vi "setTrigger.vi"(8 "error in":errorcluster, 9 "Trigger Settings":T3={"DC Restore"=enum."off", "Polarity"=enum."Negative", "TV Event"=enum."Field 1", "Coupling"=enum."AC", "Slope"=enum."Negative", "AnalogSource"=enum."Channel 0", "Window Mode"=enum."Entering", "Low Level"=0.0, "High Level"=0.0, "Hysteresis"=0.0, "Delay"=0.0, "Holdoff"=0.0, "Signal Format"=enum."M-NTSC", "Mode"=enum."Immediate", "Line Number"=0, "DigitalSource"=enum."RTSI 0"}, 11 "instrument handle":refnum<k15>) -> (0 "error out":errorcluster, 1 "Trigger Settings out":T3={"DC Restore"=enum."off", "Polarity"=enum."Negative", "TV Event"=enum."Field 1", "Coupling"=enum."AC", "Slope"=enum."Negative", "AnalogSource"=enum."Channel 0", "Window Mode"=enum."Entering", "Low Level"=0.0, "High Level"=0.0, "Hysteresis"=0.0, "Delay"=0.0, "Holdoff"=0.0, "Signal Format"=enum."M-NTSC", "Mode"=enum."Immediate", "Line Number"=0, "DigitalSource"=enum."RTSI 0"}, 3 "instrument handle out":refnum<k15>)   [LabVIEW 2011]
uses:
  niScope trigger source.ctl
  niScope trigger source digital.ctl
  TriggerSettings_TypDef.ctl
  OnOffTypeDef.ctl
  Polarity_TypDEf.ctl
  TVEvent_TypDef.ctl
  coupling_TypDef.ctl
  positive_negatice2_typDef.ctl
  TriggerSource_TypDef.ctl
  triggerwindowmode2_TypDef.ctl
  SignalFormat_TypDef.ctl
  mode_TypDef.ctl
  Trigger.DigitalSource_TypDEf.ctl
  LVStringsAndValuesArrayTypeDef.ctl
panel:
  in  "Trigger Source window 2":T1="0" caption="Source"
  out "Channel Selection out":string
  out "Mode":T2
  in  "trigger source (dig)":T13="VAL_RTSI_0" caption="trigger source (RTSI 0)"
  in  "Trigger Source Video 2":T1="0" caption="Source"
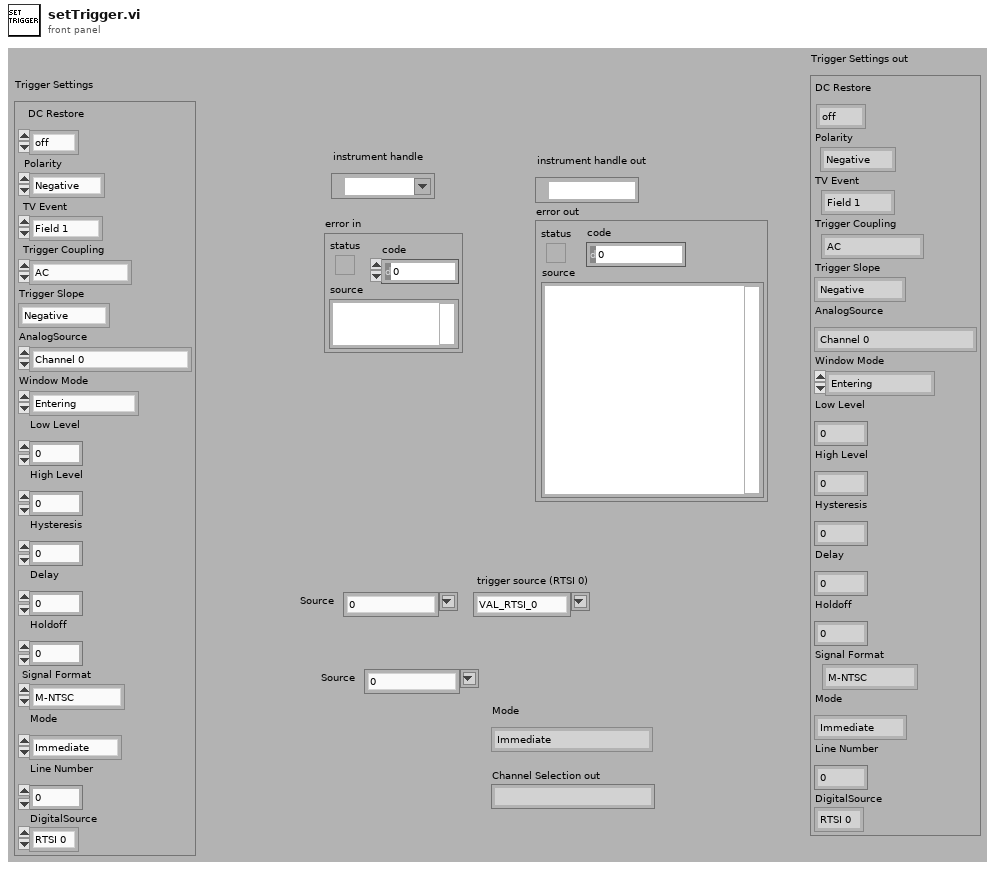
[diagram p1: front panel]
types:
  T1 = typedef "niScope trigger source.ctl" = string
  T2 = typedef "mode_TypDef.ctl" = enum32{"Immediate", "Analog Edge", "Analog Window", "Analog Hysteresis", "Video", "Digital Edge"}
  T3 = typedef "TriggerSettings_TypDef.ctl" = cluster{"DC Restore":T4, "Polarity":T5, "TV Event":T6, "Coupling":T7, "Slope":T8, "AnalogSource":T9, "Window Mode":T10, "Low Level":dbl, "High Level":dbl, "Hysteresis":dbl, "Delay":dbl, "Holdoff":dbl, "Signal Format":T11, "Mode":T2, "Line Number":i32, "DigitalSource":T12}
  T4 = typedef "OnOffTypeDef.ctl" = enum16{"off", "on"}
  T5 = typedef "Polarity_TypDEf.ctl" = enum16{"Negative", "Positive"}
  T6 = typedef "TVEvent_TypDef.ctl" = enum16{"Field 1", "Field 2", "Any Field", "Any Line", "Line Number"}
  T7 = typedef "coupling_TypDef.ctl" = enum16{"AC", "DC", "HF Reject", "LF Reject", "AC Plus HF Reject"}
  T8 = typedef "positive_negatice2_typDef.ctl" = enum16{"Positive", "Negative"}
  T9 = typedef "TriggerSource_TypDef.ctl" = enum16{"Channel 0", "Channel 1", "External TRIG"}
  T10 = typedef "triggerwindowmode2_TypDef.ctl" = enum16{"Entering", "Leaving"}
  T11 = typedef "SignalFormat_TypDef.ctl" = enum16{"M-NTSC", "B/G-PAL", "SECAM", "M-PAL", "480i/59.94 fps", "480i/60 fps", "480p/59.94 Fps", "480p/60 Fps", "576i/50 fps", "576p/50 Fps", "720p/50 Fps", "720p/59.94 Fps", "720p/60 Fps", "1080i/50 fps", "1080i/59.94 fps", "1080i/60 fps", "1080p/24 Fps"}
  T12 = typedef "Trigger.DigitalSource_TypDEf.ctl" = enum16{"RTSI 0", "RTSI 1", "RTSI 2", "RTSI 3", "RTSI 4", "RTSI 5", "RTSI 6", "PFI 0", "PFI 1", "PFI 2", "PXI Star Trigger"}
  T13 = typedef "niScope trigger source digital.ctl" = string
  T14 = typedef "LVStringsAndValuesArrayTypeDef.ctl" = cluster{"String":string, "Value":ext}[]
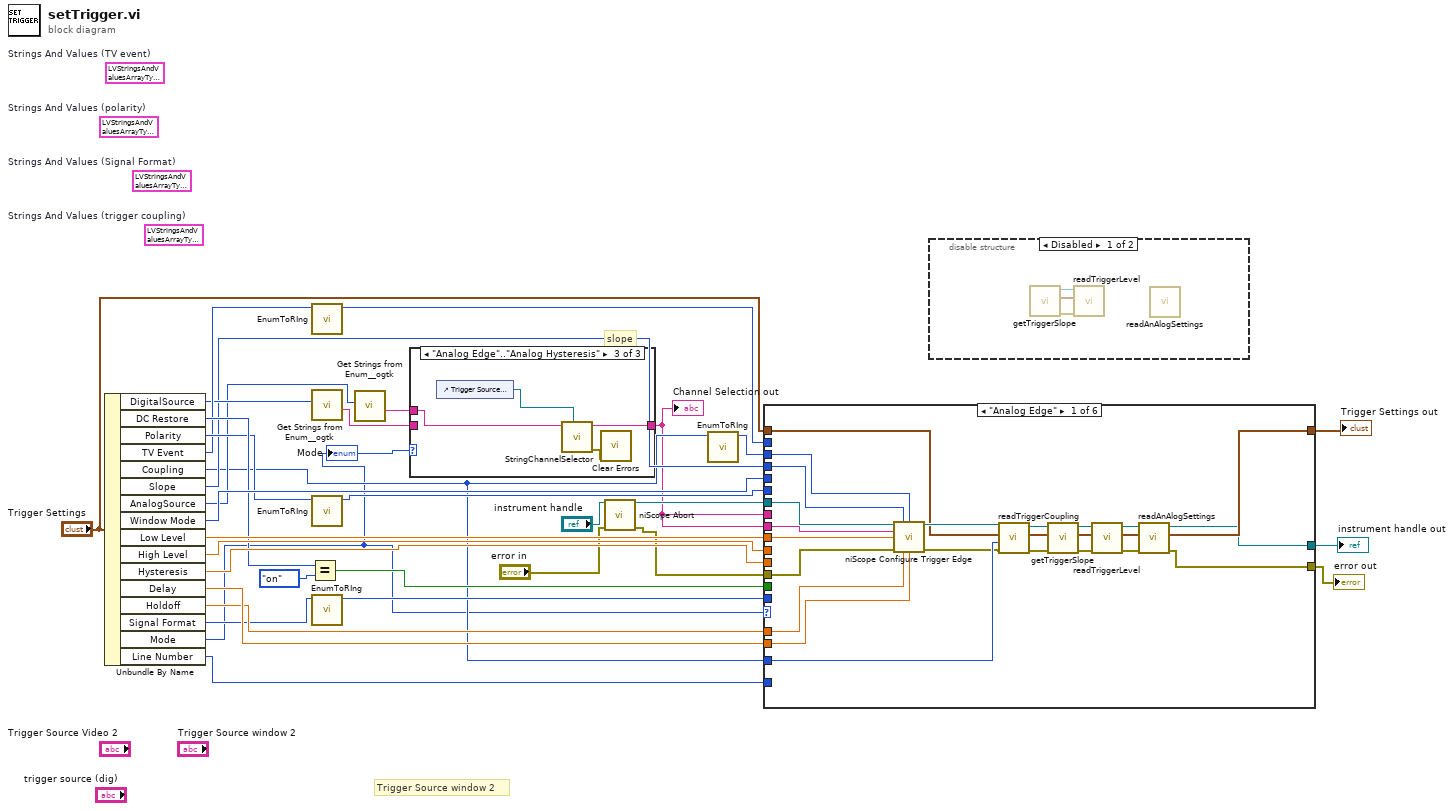
[diagram p0: block diagram]
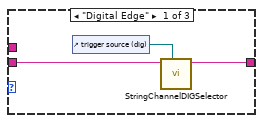
[diagram p3: hidden frame]
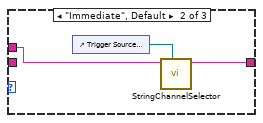
[diagram p4: hidden frame]
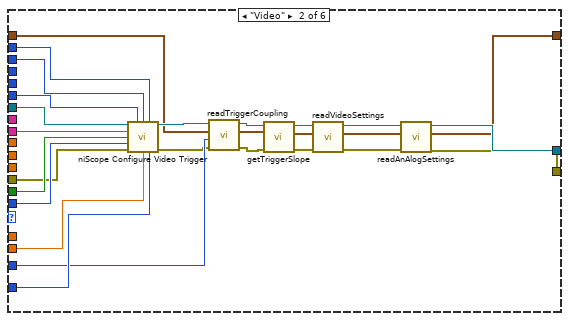
[diagram p5: hidden frame]
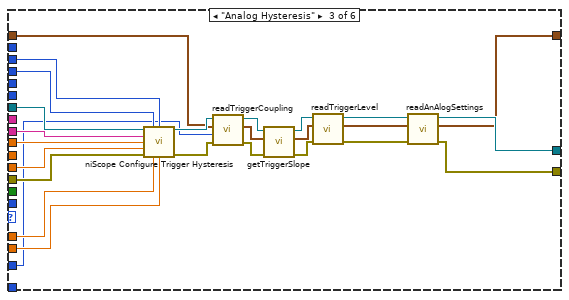
[diagram p6: hidden frame]
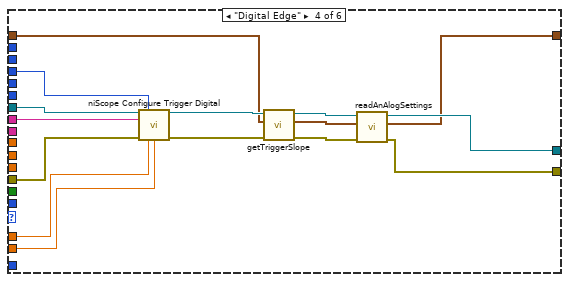
[diagram p7: hidden frame]
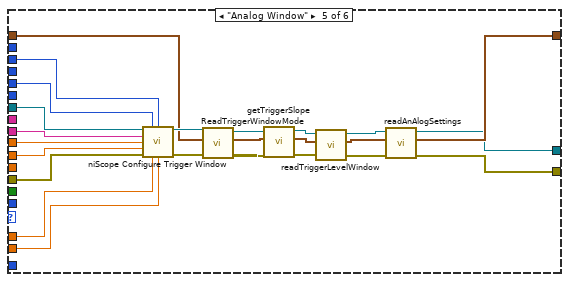
[diagram p8: hidden frame]
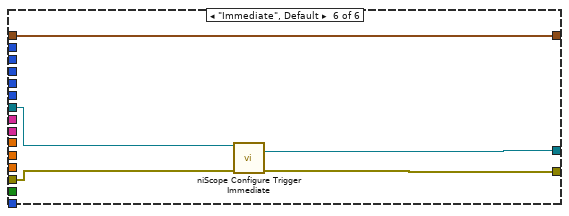
[diagram p9: hidden frame]
diagram:
  (unwired) T14 [{"String"="M-NTSC", "Value"=1.0}, {"String"="B/G-PAL", "Value"=2.0}, {"String"="SECAM", "Value"=3.0}, {"String"="M-PAL", "Value"=1001.0}, {"String"="480i/59.94 fps", "Value"=1010.0}, {"String"="480i/60 fps", "Value"=1011.0}, {"String"="480p/59.94 Fps", "Value"=1015.0}, {"String"="480p/60 Fps", "Value"=1016.0}, {"String"="576i/50 fps", "Value"=1020.0}, {"String"="576p/50 Fps", "Value"=1025.0}, {"String"="720p/50 Fps", "Value"=1031.0}, {"String"="720p/59.94 Fps", "Value"=1032.0}, {"String"="720p/60 Fps", "Value"=1033.0}, {"String"="1080i/50 fps", "Value"=1040.0}, {"String"="1080i/59.94 fps", "Value"=1041.0}, {"String"="1080i/60 fps", "Value"=1042.0}, {"String"="1080p/24 Fps", "Value"=1045.0}]  # Strings And Values (Signal Format)
  (unwired) T14 [{"String"="Field 1", "Value"=1.0}, {"String"="Field 2", "Value"=2.0}, {"String"="Any Field", "Value"=3.0}, {"String"="Any Line", "Value"=4.0}, {"String"="Line Number", "Value"=5.0}]  # Strings And Values (TV event)
  (unwired) T14 [{"String"="Positive", "Value"=1.0}, {"String"="Negative", "Value"=2.0}]  # Strings And Values (polarity)
  (unwired) T14 [{"String"="AC", "Value"=0.0}, {"String"="DC", "Value"=1.0}, {"String"="HF Reject", "Value"=3.0}, {"String"="LF Reject", "Value"=4.0}, {"String"="AC Plus HF Reject", "Value"=1001.0}]  # Strings And Values (trigger coupling)
  # "Trigger Source window 2"
  # "slope"
  n1 = Unbundle By Name("Trigger Settings") -> ("DigitalSource"=w15:T12, "DC Restore"=w26:T4, "Polarity"=w18:T5, "TV Event"=w17:T6, "Coupling"=w7:T7, "Slope"=w11:T8, "AnalogSource"=w8:T9, "Window Mode"=w33:T10, "Low Level"=w32:dbl, "High Level"=w31:dbl, "Hysteresis"=w30:dbl, "Delay"=w29:dbl, "Holdoff"=w28:dbl, "Signal Format"=w16:T11, "Mode"=w5:T2, "Line Number"=w27:i32)
  "Mode" <- w5
  n2 = Equal?(x=w26, y=OnOffTypeDef."on" ("DC Restore")) -> (x = y?=w24:bool)
  n3 = call "EnumToRIng.vi"("Enum"=w17) -> ("Ring (Value)"=w21:u16)  [unwired: 10 in]
  n4 = call "Get Strings from Enum__ogtk.vi"("Enum"=w15) -> ("String Value"=w14:string)  [unwired: 7 in, 3 out]
  n5 = call "EnumToRIng.vi"("Enum"=w18) -> ("Ring (Value)"=w22:u16)  [unwired: 10 in]
  n6 = call "EnumToRIng.vi"("Enum"=w16) -> ("Ring (Value)"=w19:u16)  [unwired: 10 in]
  n7 = call "Get Strings from Enum__ogtk.vi"("Enum"=w8) -> ("String Value"=w23:string)  [unwired: 7 in, 3 out]
  n8 = case shown="\"Analog Edge\"..\"Analog Hysteresis\"" w5 {
    tunnel: [w35 w38 w43] -> w3
    tunnel: w23 -> [_ w37 w42]
    tunnel: w14 -> [w34 _ _]
    frame "Digital Edge" {
      n9 = control-ref of="trigger source (dig)"() -> (w36:refnum<vi>)
      n10 = call "StringChannelDIGSelector.vi"("ComboBoxREF"=w36, "input string"=w34) -> ("trigger source (dig)"=w35:T13)  [unwired: 8 in, 1 out]
    }
    frame "Immediate", Default {
      n11 = control-ref of="Trigger Source Video 2"() -> (w39:refnum<vi>)
      n12 = call "StringChannelSelector.vi"("reference 2"=w39, "input string"=w37) -> ("Channel Selection out"=w38:string)  [unwired: 8 in, 1 out]
    }
    frame "Analog Edge".."Analog Hysteresis" {
      n13 = control-ref of="Trigger Source window 2"() -> (w41:refnum<vi>)
      n14 = call "StringChannelSelector.vi"("reference 2"=w41, "input string"=w42) -> ("error out"=w40:errorcluster, "Channel Selection out"=w43:string)  [unwired: 8 in]
      n15 = call "Clear Errors.vi"("error in (no error)"=w40) -> ()  [unwired: 6 in, 1 out]
    }
  }
  "Channel Selection out" <- w3
  n16 = call "niScope Abort.vi"("instrument handle"="instrument handle", "error in"="error in") -> ("instrument handle out"=w12:refnum<k15>, "error out"=w1:errorcluster)  [unwired: 12 in]
  n17 = call "EnumToRIng.vi"("Enum"=w7) -> ("Ring (Value)"=w20:u16)  [unwired: 10 in]
  n18 = case "Trigger Selection" shown="\"Analog Edge\"" w5 {
    tunnel: [w46 w68 w94 w119 w146 w161] -> w6
    tunnel: [w58 w72 w108 w121 w147 w162] -> w10
    tunnel: w29 -> [w67 w93 w118 w133 w157 _]
    tunnel: w20 -> [w66 w92 w117 _ w156 _]
    tunnel: w11 -> [w57 _ w116 w132 _ _]
    tunnel: w32 -> [w61 _ w115 _ w155 _]
    tunnel: w3 -> [w65 w91 w114 _ w154 _]
    tunnel: w3 -> [_ _ _ w131 _ _]
    tunnel: w12 -> [w64 w90 w113 w130 w153 w160]
    tunnel: w28 -> [w63 _ w112 w129 w152 _]
    tunnel: w31 -> [_ _ _ _ w151 _]
    tunnel: w33 -> [_ _ _ _ w150 _]
    tunnel: w21 -> [_ w84 _ _ _ _]
    tunnel: w22 -> [_ w89 _ _ _ _]
    tunnel: w24 -> [_ w88 _ _ _ _]
    tunnel: w19 -> [_ w87 _ _ _ _]
    tunnel: w27 -> [_ w86 _ _ _ _]
    tunnel: w30 -> [_ _ w111 _ _ _]
    tunnel: w1 -> [w62 w85 w110 w128 w149 w159]
    tunnel: "Trigger Settings" -> [w50 w79 w101 w125 w141 w158]
    tunnel: [w59 w70 w106 w120 w148 w158] -> w9
    tunnel: w7 -> [w53 w76 w98 _ _ _]
    frame "Analog Edge" {
      n19 = call "niScope Configure Trigger Edge.vi"("instrument handle"=w64, "trigger slope"=w57, "trigger coupling"=w66, "trigger source"=w65, "trigger level"=w61, "error in"=w62, "trigger holdoff"=w63, "trigger delay"=w67) -> ("instrument handle out"=w54:refnum<k15>, "error out"=w45:errorcluster)  [unwired: 6 in]
      n20 = call "readTriggerCoupling.vi"("error in (no error)"=w45, "Coupling"=w53, "output cluster out"=w50, "IVI Refnum in"=w54) -> ("error out"=w44:errorcluster, "output cluster"=w49:T3, "IVI Refnum out"=w51:refnum<k15>)  [unwired: 5 in]
      n21 = call "getTriggerSlope.vi"("error in (no error)"=w44, "Trigger Settings"=w49, "IVI Refnum in"=w51) -> ("error out"=w48:errorcluster, "Trigger Settings out"=w55:T3, "IVI Refnum out"=w56:refnum<k15>)  [unwired: 6 in]
      n22 = call "readTriggerLevel.vi"("error in (no error)"=w48, "output cluster in"=w55, "IVI Refnum in"=w56) -> ("error out"=w47:errorcluster, "output cluster out"=w52:T3, "IVI Refnum out"=w60:refnum<k15>)  [unwired: 6 in]
      n23 = call "readAnAlogSettings.vi"("error in (no error)"=w47, "output cluster in"=w52, "IVI Refnum in"=w60) -> ("error out"=w46:errorcluster, "output cluster out"=w59:T3, "IVI Refnum out"=w58:refnum<k15>)  [unwired: 6 in]
    }
    frame "Video" {
      n24 = call "niScope Configure Video Trigger.vi"("instrument handle"=w90, "polarity"=w89, "trigger coupling"=w92, "TV event"=w84, "trigger source"=w91, "enable DC restore"=w88, "signal format"=w87, "error in"=w85, "trigger delay"=w93, "line number"=w86) -> ("instrument handle out"=w80:refnum<k15>, "error out"=w75:errorcluster)  [unwired: 4 in]
      n25 = call "readTriggerCoupling.vi"("error in (no error)"=w75, "Coupling"=w76, "output cluster out"=w79, "IVI Refnum in"=w80) -> ("error out"=w74:errorcluster, "output cluster"=w77:T3, "IVI Refnum out"=w78:refnum<k15>)  [unwired: 5 in]
      n26 = call "getTriggerSlope.vi"("error in (no error)"=w74, "Trigger Settings"=w77, "IVI Refnum in"=w78) -> ("error out"=w81:errorcluster, "Trigger Settings out"=w83:T3, "IVI Refnum out"=w82:refnum<k15>)  [unwired: 6 in]
      n27 = call "readVideoSettings.vi"("error in (no error)"=w81, "Trigger Settings"=w83, "IVI Refnum in"=w82) -> ("error out"=w69:errorcluster, "output cluster"=w71:T3, "IVI Refnum out"=w73:refnum<k15>)  [unwired: 6 in]
      n28 = call "readAnAlogSettings.vi"("error in (no error)"=w69, "output cluster in"=w71, "IVI Refnum in"=w73) -> ("error out"=w68:errorcluster, "output cluster out"=w70:T3, "IVI Refnum out"=w72:refnum<k15>)  [unwired: 6 in]
    }
    frame "Analog Hysteresis" {
      n29 = call "niScope Configure Trigger Hysteresis.vi"("instrument handle"=w113, "trigger slope"=w116, "trigger coupling"=w117, "trigger source"=w114, "trigger level"=w115, "hysteresis"=w111, "error in"=w110, "trigger holdoff"=w112, "trigger delay"=w118) -> ("instrument handle out"=w103:refnum<k15>, "error out"=w99:errorcluster)  [unwired: 5 in]
      n30 = call "readTriggerCoupling.vi"("error in (no error)"=w99, "Coupling"=w98, "output cluster out"=w101, "IVI Refnum in"=w103) -> ("error out"=w97:errorcluster, "output cluster"=w100:T3, "IVI Refnum out"=w102:refnum<k15>)  [unwired: 5 in]
      n31 = call "getTriggerSlope.vi"("error in (no error)"=w97, "Trigger Settings"=w100, "IVI Refnum in"=w102) -> ("error out"=w96:errorcluster, "Trigger Settings out"=w104:T3, "IVI Refnum out"=w105:refnum<k15>)  [unwired: 6 in]
      n32 = call "readTriggerLevel.vi"("error in (no error)"=w96, "output cluster in"=w104, "IVI Refnum in"=w105) -> ("error out"=w95:errorcluster, "output cluster out"=w107:T3, "IVI Refnum out"=w109:refnum<k15>)  [unwired: 6 in]
      n33 = call "readAnAlogSettings.vi"("error in (no error)"=w95, "output cluster in"=w107, "IVI Refnum in"=w109) -> ("error out"=w94:errorcluster, "output cluster out"=w106:T3, "IVI Refnum out"=w108:refnum<k15>)  [unwired: 6 in]
    }
    frame "Digital Edge" {
      n34 = call "niScope Configure Trigger Digital.vi"("instrument handle"=w130, "trigger slope"=w132, "trigger source"=w131, "error in"=w128, "trigger holdoff"=w129, "trigger delay"=w133) -> ("instrument handle out"=w127:refnum<k15>, "error out"=w126:errorcluster)  [unwired: 8 in]
      n35 = call "getTriggerSlope.vi"("error in (no error)"=w126, "Trigger Settings"=w125, "IVI Refnum in"=w127) -> ("error out"=w122:errorcluster, "Trigger Settings out"=w123:T3, "IVI Refnum out"=w124:refnum<k15>)  [unwired: 6 in]
      n36 = call "readAnAlogSettings.vi"("error in (no error)"=w122, "output cluster in"=w123, "IVI Refnum in"=w124) -> ("error out"=w119:errorcluster, "output cluster out"=w120:T3, "IVI Refnum out"=w121:refnum<k15>)  [unwired: 6 in]
    }
    frame "Analog Window" {
      n37 = call "niScope Configure Trigger Window.vi"("instrument handle"=w153, "trigger window mode"=w150, "trigger coupling"=w156, "trigger source"=w154, "low level"=w155, "high level"=w151, "error in"=w149, "trigger holdoff"=w152, "trigger delay"=w157) -> ("instrument handle out"=w145:refnum<k15>, "error out"=w143:errorcluster)  [unwired: 5 in]
      n38 = call "ReadTriggerWindowMode.vi"("error in (no error)"=w143, "Trigger Settings in"=w141, "IVI Refnum in"=w145) -> ("error out"=w142:errorcluster, "Trigger Settings out"=w140:T3, "IVI Refnum out"=w144:refnum<k15>)  [unwired: 6 in]
      n39 = call "getTriggerSlope.vi"("error in (no error)"=w142, "Trigger Settings"=w140, "IVI Refnum in"=w144) -> ("error out"=w136:errorcluster, "Trigger Settings out"=w137:T3, "IVI Refnum out"=w139:refnum<k15>)  [unwired: 6 in]
      n40 = call "readTriggerLevelWindow.vi"("error in (no error)"=w136, "output cluster in"=w137, "IVI Refnum in"=w139) -> ("error out"=w134:errorcluster, "output cluster out"=w135:T3, "IVI Refnum out"=w138:refnum<k15>)  [unwired: 6 in]
      n41 = call "readAnAlogSettings.vi"("error in (no error)"=w134, "output cluster in"=w135, "IVI Refnum in"=w138) -> ("error out"=w146:errorcluster, "output cluster out"=w148:T3, "IVI Refnum out"=w147:refnum<k15>)  [unwired: 6 in]
    }
    frame "Immediate", Default {
      n42 = call "niScope Configure Trigger Immediate.vi"("instrument handle"=w160, "error in"=w159) -> ("instrument handle out"=w162:refnum<k15>, "error out"=w161:errorcluster)  [unwired: 12 in]
    }
  }
  "instrument handle out" <- w10
  "Trigger Settings out" <- w9
  "error out" <- w6
  n43 = disable-structure shown="Disabled" {
    frame Disabled {
      n44 = call "getTriggerSlope.vi"() -> ("error out"=w165:errorcluster, "Trigger Settings out"=w164:T3, "IVI Refnum out"=w163:refnum<k15>)  [unwired: 9 in]
      n45 = call "readTriggerLevel.vi"("error in (no error)"=w165, "output cluster in"=w164, "IVI Refnum in"=w163) -> ()  [unwired: 6 in, 3 out]
      n46 = call "readAnAlogSettings.vi"() -> ()  [unwired: 9 in, 3 out]
    }
    frame Enabled {
    }
  }
